vi "Write.vi"(8 "error in (no error)":errorcluster, 10 "Waveform":waveform(dbl), 11 "Abs_Waveform in":refnum<class "Abs_Waveform.lvclass">) -> (0 "error out":errorcluster, 3 "Abs_Waveform out":refnum<class "Abs_Waveform.lvclass">)   [LabVIEW 2021, in "Abs_Waveform.lvclass"]
uses:
  Abs_Waveform.lvclass
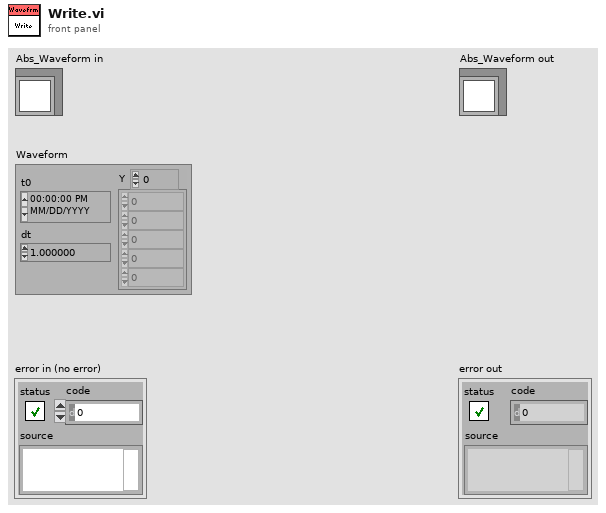
[diagram p1: front panel]
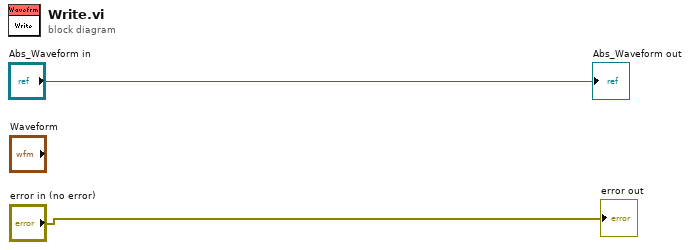
[diagram p0: block diagram]
diagram:
  "error out" <- "error in (no error)"
  "Abs_Waveform out" <- "Abs_Waveform in"
